vi "Parse.vi"(8 "Error In":errorcluster, 11 "object in":refnum<class "2021_14.lvclass">) -> (0 "Error Out":errorcluster, 3 "object out":refnum<class "2021_14.lvclass">)   [LabVIEW 2020, in "2021_14.lvclass"]
uses:
  2021_14.lvclass
  2021_14.lvclass/2021_14.ctl
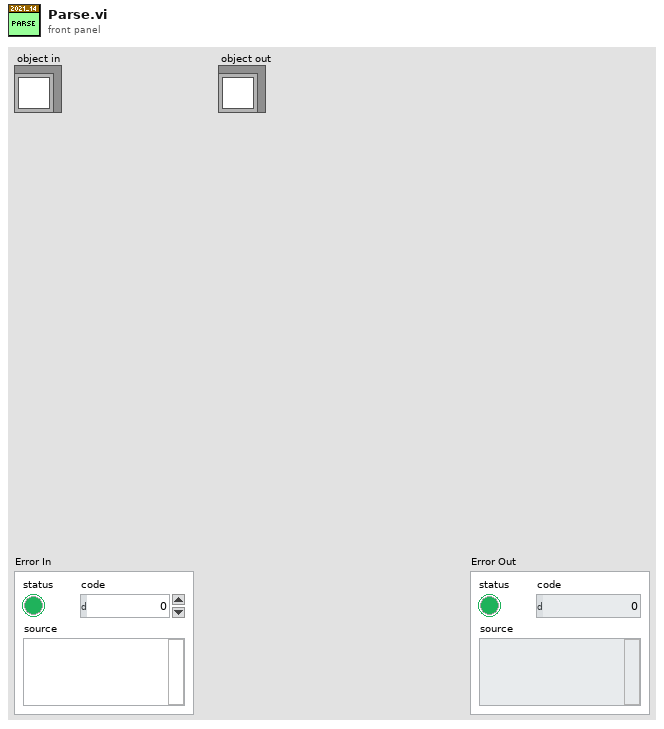
[diagram p1: front panel]
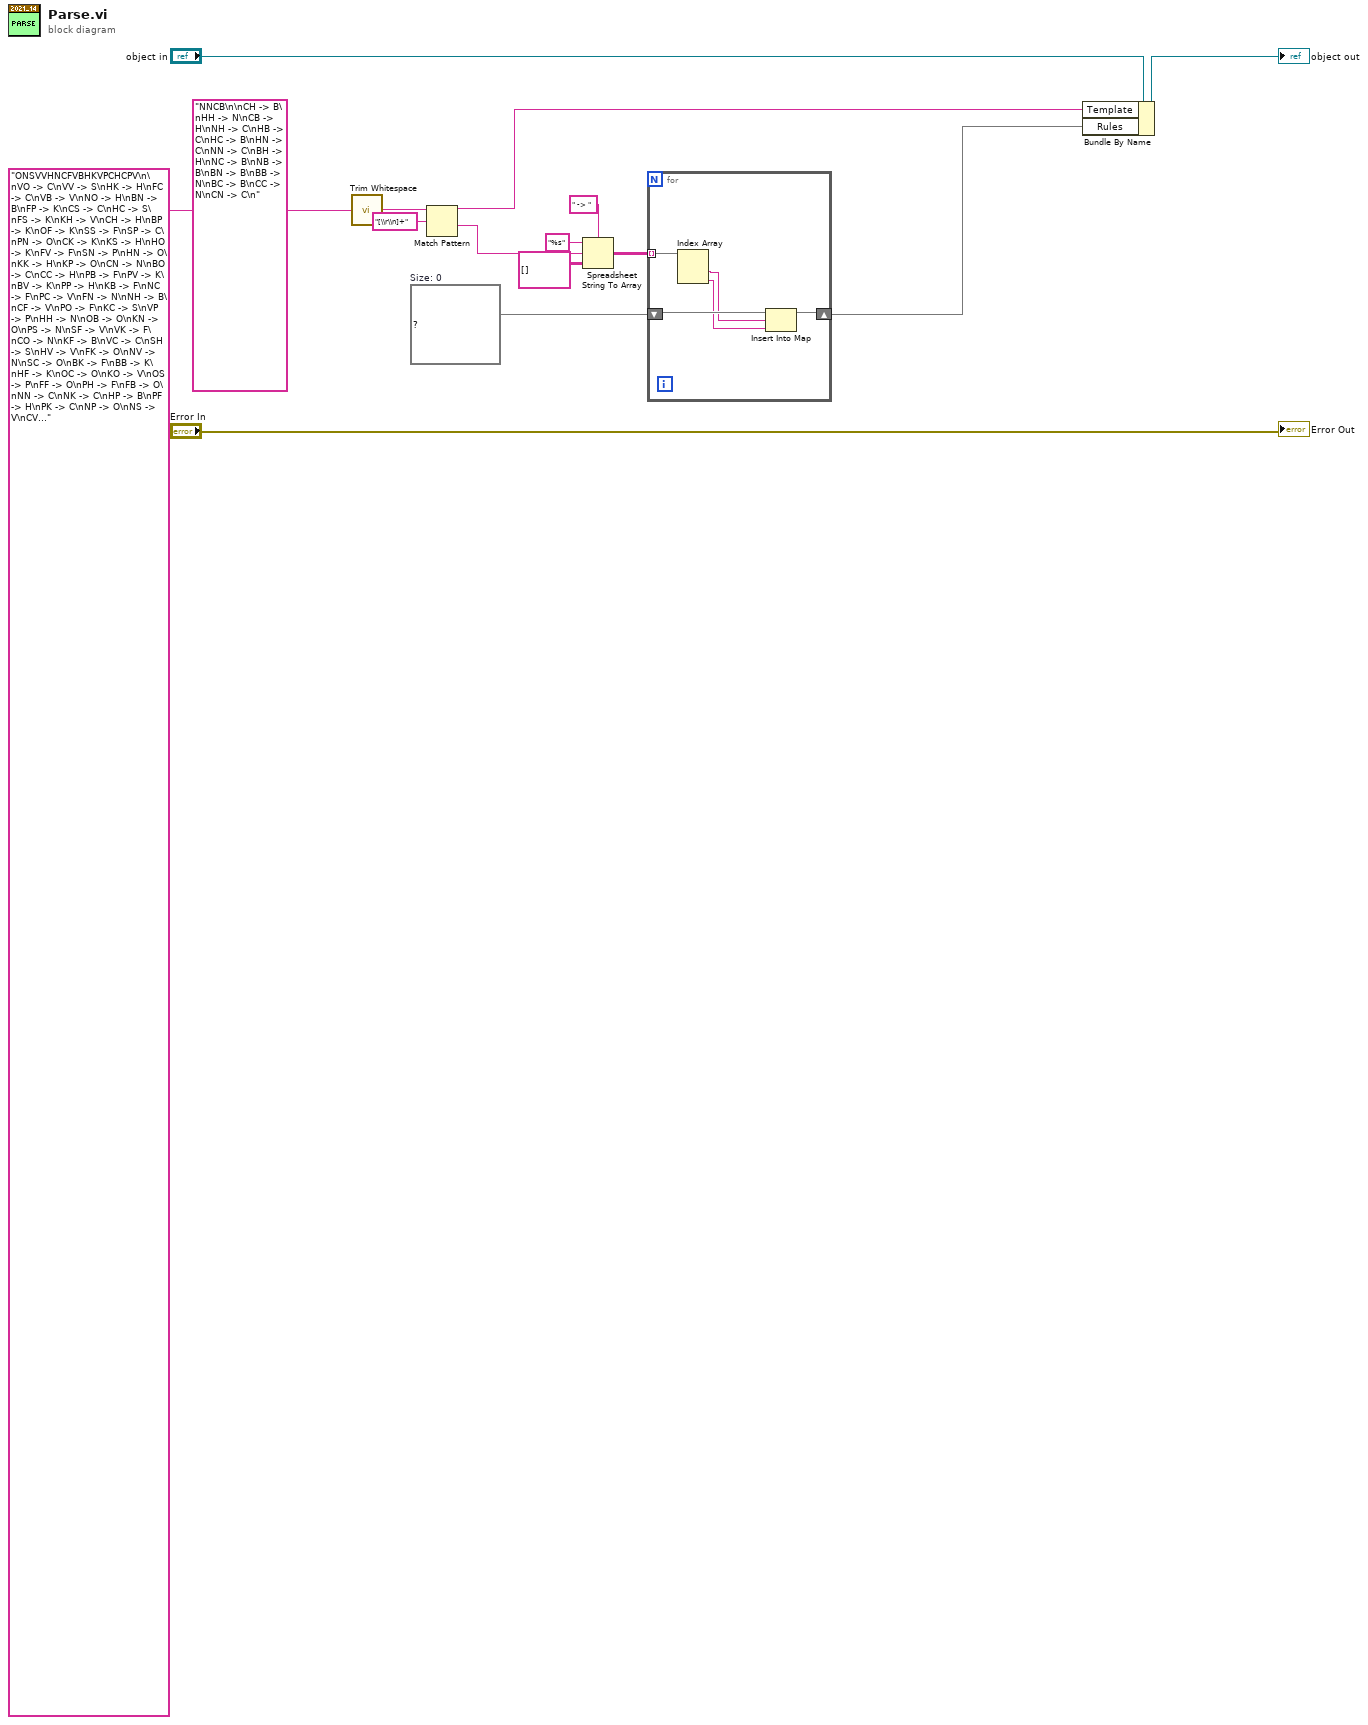
[diagram p0: block diagram]
diagram:
  w3 = map{string, string} {}  # Size: 0
  (unwired) "NNCB\n\nCH -> B\nHH -> N\nCB -> H\nNH -> C\nHB -> C\nHC -> B\nHN -> C\nNN -> C\nBH -> H\nNC -> B\nNB -> B\nBN -> B\nBB -> N\nBC -> B\nCC -> N\nCN -> C\n" ("regular expression")
  n1 = call <vilib>:"Trim Whitespace.vi"("string"="ONSVVHNCFVBHKVPCHCPV\n\nVO -> C\nVV -> S\nHK -> H\nFC -> C\nVB -> V\nNO -> H\nBN -> B\nFP -> K\nCS -> C\nHC -> S\nFS -> K\nKH -> V\nCH -> H\nBP -> K\nOF -> K\nSS -> F\nSP -> C\nPN -> O\nCK -> K\nKS -> H\nHO -> K\nFV -> F\nSN -> P\nHN -> O\nKK -> H\nKP -> O\nCN -> N\nBO -> C\nCC -> H\nPB -> F\nPV -> K\nBV -> K\nPP -> H\nKB -> F\nNC -> F\nPC -> V\nFN -> N\nNH -> B\nCF -> V\nPO -> F\nKC -> S\nVP -> P\nHH -> N\nOB -> O\nKN -> O\nPS -> N\nSF -> V\nVK -> F\nCO -> N\nKF -> B\nVC -> C\nSH -> S\nHV -> V\nFK -> O\nNV -> N\nSC -> O\nBK -> F\nBB -> K\nHF -> K\nOC -> O\nKO -> V\nOS -> P\nFF -> O\nPH -> F\nFB -> O\nNN -> C\nNK -> C\nHP -> B\nPF -> H\nPK -> C\nNP -> O\nNS -> V\nCV -> O\nVH -> C\nOP -> N\nSO -> O\nSK -> H\nSV -> O\nNF -> H\nBS -> K\nBH -> O\nVN -> S\nHB -> O\nOH -> K\nCB -> B\nBC -> S\nOV -> F\nBF -> P\nOO -> F\nHS -> H\nON -> P\nNB -> F\nCP -> S\nSB -> V\nVF -> C\nOK -> O\nFH -> H\nKV -> S\nFO -> C\nVS -> B\n" ("PuzzleInput")) -> ("trimmed string"=w8:string)  [unwired: 1 in]
  n2 = Match Pattern(string=w8, regular expression="[\\r\\n]+") -> (before substring=w5:string, after substring=w6:string)  [unwired: 1 in, 2 out]
  n3 = Spreadsheet String To Array(delimiter (Tab)=" -> ", format string="%s", spreadsheet string=w6, array type (2D Dbl)=string[][] []) -> (array=w4:string[][])
  n4 = for {
    tunnel: w4 -> [w19] mode=indexing
    shift-right: [w17] -> w2
    shift-left: w3 -> [w18]
    n5 = Index Array(array=w19) -> (element #1=w16:string, element #2=w15:string)  [unwired: 2 in]
    n6 = Insert Into Map(map in=w18, key=w16, value=w15) -> (map out=w17:map{string, string})  [unwired: 2 out]
  }
  n7 = Bundle By Name(cluster="object in", "Template"=w5, "Rules"=w2) -> (→"object out":refnum<class "2021_14.lvclass">)
  "Error Out" <- "Error In"
